vi "Open.vi"(8 "error in (no error)":errorcluster, 11 "PythonWrapper in":refnum<class "PythonWrapper.lvclass">) -> (0 "error out":errorcluster, 3 "PythonWrapper out":refnum<class "PythonWrapper.lvclass">)   [LabVIEW 2022 SP3, in "PythonWrapper.lvlib" / "PythonWrapper.lvclass"]
uses:
  PythonWrapper.lvclass
  PythonWrapper.lvclass/PythonWrapper.ctl
  PythonSession/PythonSession.lvclass
  PathUtils/Source/PathUtils.lvlib
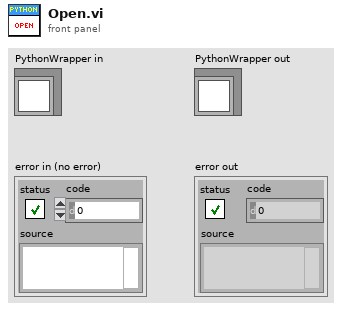
[diagram p1: front panel]
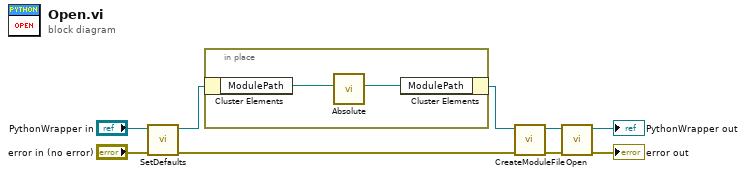
[diagram p0: block diagram]
diagram:
  n1 = call-dynamic "SetDefaults.vi"("error in (no error)"="error in (no error)", "PythonWrapper in"="PythonWrapper in") -> ("error out"=w6:errorcluster, "PythonWrapper out"=w4:refnum<class "PythonWrapper.lvclass">)  [unwired: 8 in]
  n2 = in-place {
    n3 = in-place-cluster #1(w4) -> ("ModulePath"=w11:path)
    n4 = call "Absolute.vi"("Path in"=w11) -> ("Path out"=w10:path)  [unwired: 10 in]
    n5 = in-place-cluster #1("ModulePath"=w10) -> (w2:refnum<class "PythonWrapper.lvclass">)
  }
  n6 = call-dynamic "CreateModuleFile.vi"("error in (no error)"=w6, "PythonWrapper in"=w2) -> ("error out"=w3:errorcluster, "PythonWrapper out"=w1:refnum<class "PythonWrapper.lvclass">)  [unwired: 8 in]
  n7 = call-parent "Open.vi"("error in (no error)"=w3, "PythonSession in"=w1) -> ("error out"=→"error out":errorcluster, "PythonSession out"=→"PythonWrapper out":refnum<class "PythonWrapper.lvclass">)  [unwired: 8 in]
